vi "opposite.vi"(1 "x 2":enum32{"Current", "Voltage"}(ring)=enum."Voltage") -> (0 "x":enum32{"Current", "Voltage"}(ring))   [LabVIEW 2025, in "MySMU.lvlib"]
uses:
  MySMU.lvlib
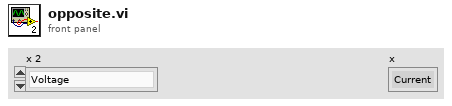
[diagram p1: front panel]
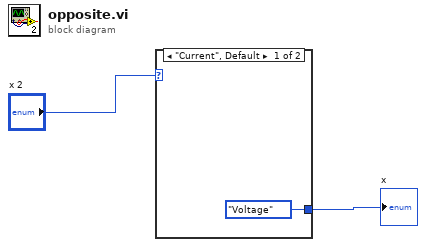
[diagram p0: block diagram]
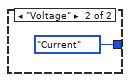
[diagram p2: hidden frame]
diagram:
  n1 = case shown="\"Current\", Default" "x 2" {
    tunnel: [enum32{"Current", "Voltage"}."Voltage" ("x") enum32{"Current", "Voltage"}."Current" ("x")] -> w1
    frame "Current", Default {
    }
    frame "Voltage" {
    }
  }
  "x" <- w1
